vi "Write Integer.vi"(8 "error in (no error)":errorcluster, 10 "Integer":i32, 11 "KDemoDerived in":refnum<class "KDemoDerived.lvclass">) -> (0 "error out":errorcluster, 3 "KDemoDerived out":refnum<class "KDemoDerived.lvclass">)   [LabVIEW 2015, in "KDemoDerived.lvclass"]
uses:
  KDemoDerived.lvclass
  KDemoDerived.lvclass/KDemoDerived.ctl
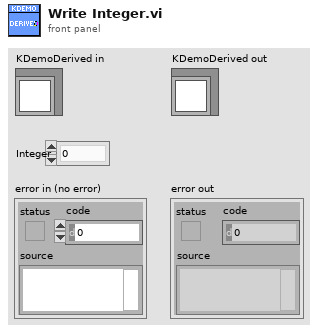
[diagram p1: front panel]
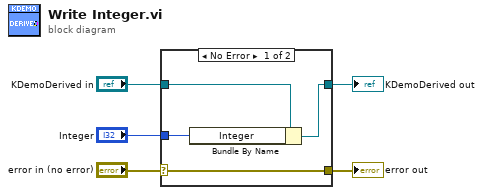
[diagram p0: block diagram]
diagram:
  n1 = case shown="No Error" "error in (no error)" {
    selector: "error in (no error)" -> [w9 w10]
    tunnel: [w9 w10] -> w4
    tunnel: [w7 w11] -> w2
    tunnel: "KDemoDerived in" -> [w8 w11]
    tunnel: "Integer" -> [w6 _]
    frame No Error {
      n2 = Bundle By Name(cluster=w8, "Integer"=w6) -> (w7:refnum<class "KDemoDerived.lvclass">)
    }
    frame Error {
    }
  }
  "error out" <- w4
  "KDemoDerived out" <- w2
